vi "EasyXML Options - Default Data.vi"(8 "error in":errorcluster) -> (0 "error out":errorcluster, 3 "Default Easy XML Options":T1)   [LabVIEW 2011]
uses:
  EasyXML Options - Data Cluster.ctl
  EasyXML Options - Type Formatting Cluster.ctl
  Support/Type Defs/Formatting Data Type -- Enum.ctl
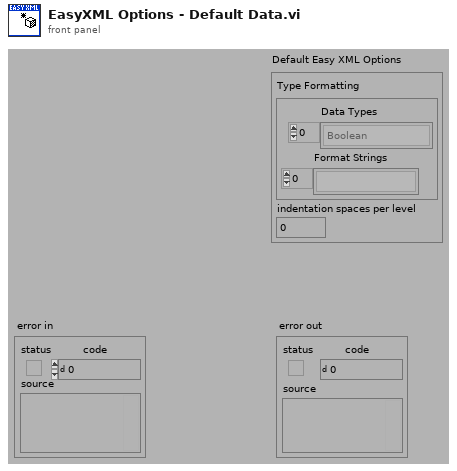
[diagram p1: front panel]
types:
  T1 = typedef "EasyXML Options - Data Cluster.ctl" = cluster{"Type Formatting":T2, "indentation spaces per level":i32}
  T2 = typedef "EasyXML Options - Type Formatting Cluster.ctl" = cluster{"Data Types":T3[], "Format Strings":string[]}
  T3 = typedef "Formatting Data Type -- Enum.ctl" = enum16{"<unknown>", "Cluster", "Array", "String", "Path", "Boolean", "Time Stamp", "Enum", "Numeric - EXT", "Numeric - DBL", "Numeric - SGL", "Numeric - I64", "Numeric - I32", "Numeric - I16", "Numeric - I8", "Numeric - U64", "Numeric - U32", "Numeric - U16", "Numeric - U8", "Numeric - CXT", "Numeric - CDB", "Numeric - CSG", "VISA Resource"}
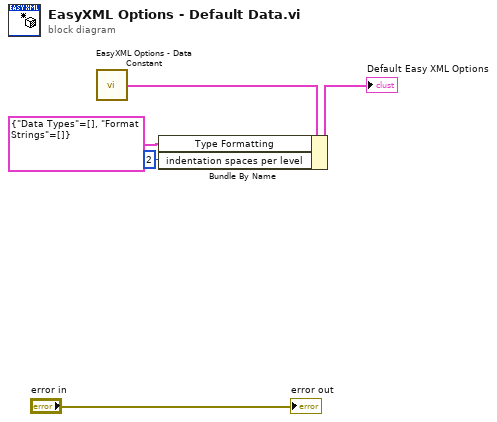
[diagram p0: block diagram]
diagram:
  n1 = call "EasyXML Options - Data Constant.vi"() -> ("Easy XML Options"=w5:T1)
  n2 = Bundle By Name(cluster=w5, "Type Formatting"=T2 {"Data Types"=[], "Format Strings"=[]}, "indentation spaces per level"=2) -> (→"Default Easy XML Options":T1)
  "error out" <- "error in"
